vi "MathCad_Numeric_Get_Ref.vi"(3 "error in (no error)":errorcluster, 4 "Variable  Name":string, 5 "Worksheet Reference In":refnum<k7>) -> (0 "error out":errorcluster, 1 "Mathcad.INumericValue Refnum":refnum<k7>, 2 "Worksheet Reference Out":refnum<k7>)   [LabVIEW 2015]
doc: "Retrieves a reference from a Mathcad worksheet,based on the variable name. If the variable is defined more than once it is the last value in the worksheet."
panel:
  in  "Mathcad.INumericValue":refnum<k7>
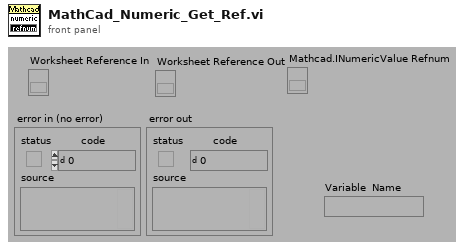
[diagram p1: front panel]
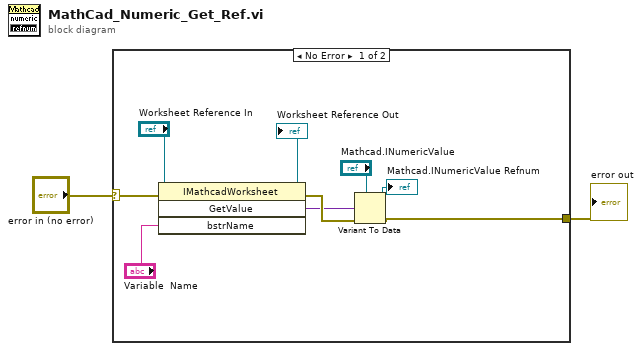
[diagram p0: block diagram]
diagram:
  n1 = case shown="No Error" "error in (no error)" {
    selector: "error in (no error)" -> [w3 w12]
    tunnel: [w11 w12] -> w2
    frame No Error {
      n2 = invoke class="IMathcadWorksheet" method="GetValue"(reference="Worksheet Reference In", error in=w3, "bstrName"="Variable  Name") -> (reference out=→"Worksheet Reference Out":refnum<k7>, error out=w9:errorcluster, "GetValue"=w8:variant)  [unwired: 1 in, 1 out]
      n3 = Variant To Data(error in=w9, type="Mathcad.INumericValue", Variant=w8) -> (data=→"Mathcad.INumericValue Refnum":refnum<k7>, error out=w11:errorcluster)
    }
    frame Error {
    }
  }
  "error out" <- w2
